vi "MacroExecTimeCalc.vi"(8 "Error In":errorcluster) -> (0 "Error Out":errorcluster, 2 "Estimated Timing cluster":T1, 3 "Estimated Time":dbl)   [LabVIEW 2012]
doc: "SciScan 1.2 160622"
uses:
  FGV_MacroCore_Commands.ctl
  Macro Loop Manager Module/SubVIs/Macro Execution and Timing_Commands.ctl
  GFG/GFG library.lvlib
  GFG/GFGnumericGet.vi
panel:
  out "Current Command":string
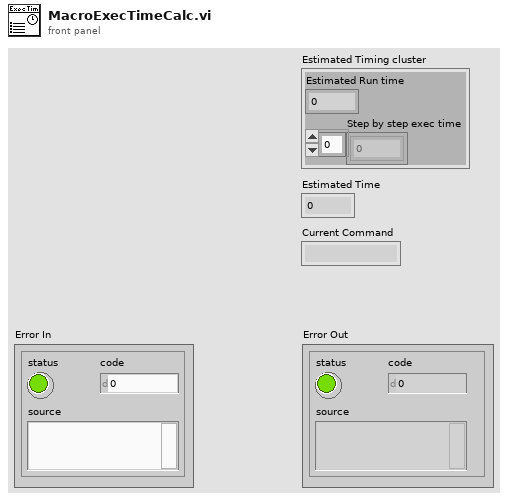
[diagram p1: front panel]
types:
  T1 = cluster{"Estimated Run time":dbl, "Step by step exec time":dbl[]}
  T2 = typedef "Macro Execution and Timing_Commands.ctl" = enum16{"Initialize (Update FGV & Rst Idx)", "Run", "EstimateTime", "Preview", "Update Macro array (Idx Unchanged)", "Update Index", "Clear Timing Info"}
  T3 = typedef "FGV_MacroCore_Commands.ctl" = enum16{"Initialize", "Get Array", "Load macro from file", "Insert Item", "Insert at End", "Edit Parameter String", "Delete instruction", "Move Items", "Save", "SaveAs", "UpdateInfoTable", "Edit Settings File", "New Macro", "Read Temp File", "Delete Multiple"}
  T4 = typedef "Estimated Timing Cluster.ctl" = cluster{"Estimated Run time":dbl, "Step by step exec time":dbl[]}
  T5 = typedef "ExecutionStatus.ctl" = enum16{"Instruction Available", "Skip", "Exec Paused", "Exec Complete", "Exec Waiting for Trigger"}
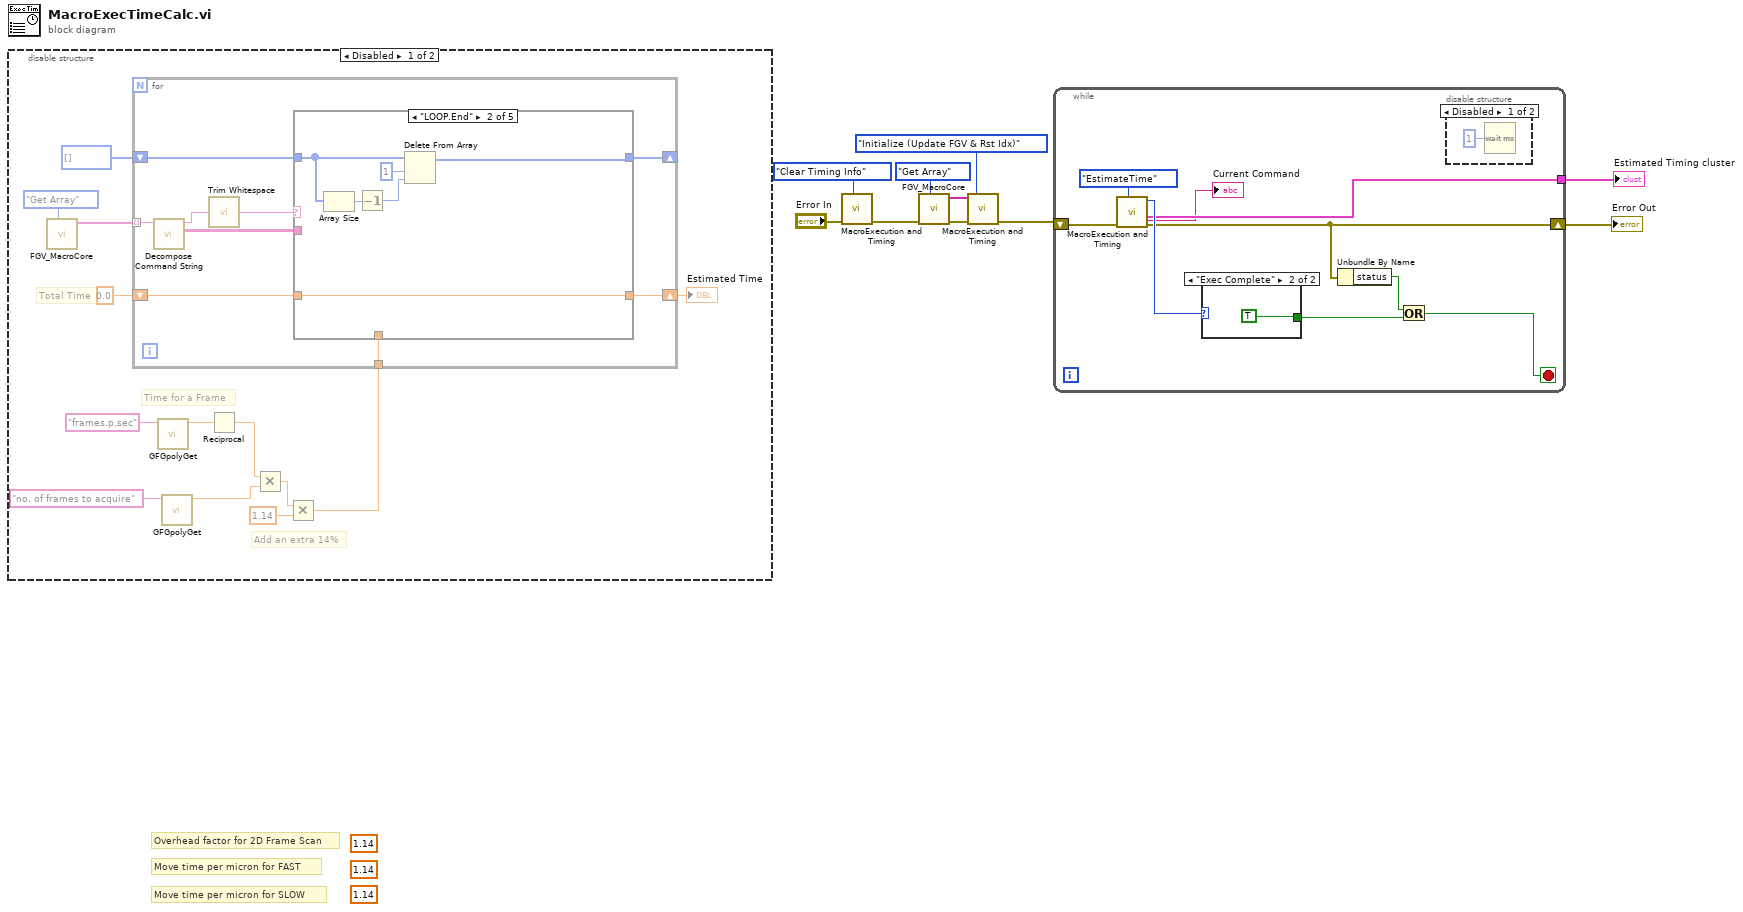
[diagram p0: block diagram]
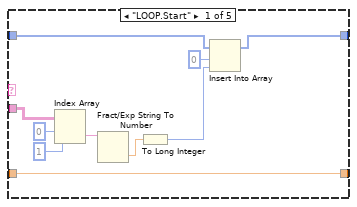
[diagram p2: hidden frame]
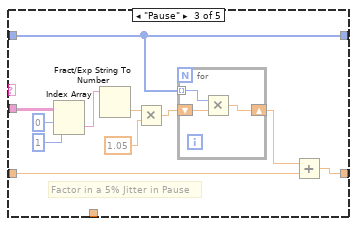
[diagram p3: hidden frame]
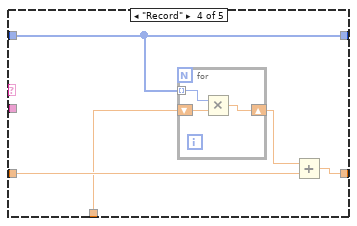
[diagram p4: hidden frame]
diagram:
  (unwired) 1.14 ("y")
  (unwired) 1.14 ("y")
  (unwired) 1.14 ("y")
  # "Move time per micron for SLOW"
  # "Move time per micron for FAST"
  # "Overhead factor for 2D Frame Scan"
  n1 = disable-structure shown="Disabled" {
    frame Disabled {
      # "Add an extra 14%"
      # "Total Time"
      # "Time for a Frame"
      n2 = call "FGV_MacroCore.vi"("MacroFGV_Commands"=FGV_MacroCore_Commands."Get Array") -> ("Macro String Array"=w18:string[])  [unwired: 6 in, 4 out]
      n3 = call-poly "GFGpolyGet.vi"("Variable Name in"="frames.p.sec") -> ("Numeric"=w21:dbl)  [unwired: 8 in, 2 out]
      n4 = call-poly "GFGpolyGet.vi"("Variable Name in"="no. of frames to acquire") -> ("Numeric"=w20:dbl)  [unwired: 8 in, 2 out]
      n5 = Reciprocal(x=w21) -> (1/x=w14:dbl)
      n6 = Multiply(x=w14, y=w20) -> (x*y=w13:dbl)
      n7 = Multiply(x=w13, y=1.14) -> (x*y=w11:dbl)
      n8 = for {
        tunnel: w18 -> [w32] mode=indexing
        tunnel: w11 -> [w24]
        shift-right: [w29] -> _
        shift-left: i32[] [] -> [w30]
        shift-right: [w25] -> w15
        shift-left: 0.0 -> [w26]
        n9 = call "Decompose Command String.vi"("Command IN"=w32) -> ("Parameter Table"=w31:string[][], "Action"=w28:string)  [unwired: 7 in, 2 out]
        n10 = call <vilib>:"Trim Whitespace.vi"("string"=w28) -> ("trimmed string"=w27:string)  [unwired: 1 in]
        n11 = case shown="\"LOOP.End\"" w27 {
          tunnel: w31 -> [w42 _ w56 _ _]
          tunnel: w30 -> [w35 w47 w55 w67 w72]
          tunnel: [w34 w44 w55 w67 w72] -> w29
          tunnel: w26 -> [w33 w43 w53 w65 w71]
          tunnel: [w33 w43 w52 w64 w71] -> w25
          tunnel: w24 -> [_ _ _ w63 _]
          frame "LOOP.Start" {
            n12 = Index Array(array=w42, index (row)=0, index (col)=1 ("disabled index (col)")) -> (element=w39:string)
            n13 = Fract/Exp String To Number(string=w39) -> (number=w38:dbl)  [unwired: 3 in, 1 out]
            n14 = To Long Integer(number=w38) -> (32bit integer=w36:i32)
            n15 = Insert Into Array(array=w35, index=0, new element=w36) -> (w34:i32[])
          }
          frame "LOOP.End" {
            n16 = Array Size(array=w47) -> (size(s)=w46:i32)
            n17 = Decrement(x=w46) -> (x-1=w45:i32)
            n18 = Delete From Array(array=w47, length=1, index=w45) -> (array with subset deleted=w44:i32[])  [unwired: 1 out]
          }
          frame "Pause" {
            # "Factor in a 5% Jitter in Pause"
            n19 = Index Array(array=w56, index (row)=0, index (col)=1 ("disabled index (col)")) -> (element=w57:string)
            n20 = Fract/Exp String To Number(string=w57) -> (number=w51:dbl)  [unwired: 3 in, 1 out]
            n21 = Multiply(x=w51, y=1.05) -> (x*y=w50:dbl)
            n22 = for {
              tunnel: w55 -> [w61] mode=indexing
              shift-right: [w60] -> w54
              shift-left: w50 -> [w62]
              n23 = Multiply(x=w61, y=w62) -> (x*y=w60:dbl)
            }
            n24 = Add(x=w54, y=w53) -> (x+y=w52:dbl)
          }
          frame "Record" {
            n25 = for {
              tunnel: w67 -> [w69] mode=indexing
              shift-right: [w68] -> w66
              shift-left: w63 -> [w70]
              n26 = Multiply(x=w69, y=w70) -> (x*y=w68:dbl)
            }
            n27 = Add(x=w66, y=w65) -> (x+y=w64:dbl)
          }
          frame Default {
          }
        }
      }
      "Estimated Time" <- w15
    }
    frame Enabled {
    }
  }
  n28 = call "MacroExecution and Timing.vi"("MacroExecution and Timing Command"=Macro_Execution_and_Timing_Commands."Clear Timing Info", "Error In"="Error In") -> ("Error Out"=w1:errorcluster)  [unwired: 4 in, 5 out]
  n29 = call "FGV_MacroCore.vi"("MacroFGV_Commands"=FGV_MacroCore_Commands."Get Array", "Error In"=w1) -> ("Error Out"=w7:errorcluster, "Macro String Array"=w6:string[])  [unwired: 5 in, 3 out]
  n30 = call "MacroExecution and Timing.vi"("MacroExecution and Timing Command"=Macro_Execution_and_Timing_Commands."Initialize (Update FGV & Rst Idx)" ("MacroExecution Command"), "Error In"=w7, "Macro IN"=w6) -> ("Error Out"=w5:errorcluster)  [unwired: 3 in, 5 out]
  n31 = while {
    shift-right: [w78] -> w4
    shift-left: w5 -> [w80]
    tunnel: [w74] -> w10
    stop <- w75 stop-if-true
    n32 = call "MacroExecution and Timing.vi"("MacroExecution and Timing Command"=Macro_Execution_and_Timing_Commands."EstimateTime" ("MacroExecution Command"), "Error In"=w80) -> ("Error Out"=w78:errorcluster, "Estimated Timing cluster"=w74:T4, "Execution Status"=w79:T5, "Current Command"=→"Current Command":string)  [unwired: 4 in, 2 out]
    n33 = case shown="\"Exec Complete\"" w79 {
      tunnel: [_ TRUE] -> w76
      frame Default {
      }
      frame "Exec Complete" {
      }
    }
    n34 = Unbundle By Name(w78) -> ("status"=w77:bool)
    n35 = Or(x=w77, y=w76) -> (x .or. y?=w75:bool)
    n36 = disable-structure shown="Disabled" {
      frame Disabled {
        n37 = Wait (ms)(milliseconds to wait=u32 1) -> ()  [unwired: 1 out]
      }
      frame Enabled {
      }
    }
  }
  "Error Out" <- w4
  "Estimated Timing cluster" <- w10
